vi "AppLauncher.vi"() -> ()   [LabVIEW 2016, in "Instrument.Example.lvclass"]
uses:
  Instrument.Example.lvclass
  <vilib>/JKI/JKI SMO/SMO/Typedefs/SMOState --Enum.ctl
  C:/Program Files (x86)/National Instruments/LabVIEW 2016/vi.lib/JKI/JKI SMO/SMO/SMO.lvclass
  C:/Program Files (x86)/National Instruments/LabVIEW 2016/user.lib/LevyLab/Levylab Instruments/SMOs/Instrument/Instrument.lvclass
  Instrument.Example UI/Instrument.Example UI.lvclass
  C:/Program Files (x86)/National Instruments/LabVIEW 2016/vi.lib/JKI/JKI SMO/SMO.UI/SMO.UI.lvclass
  <vilib>/JKI/JKI SMO/SMO/SMO.lvclass
  <vilib>/JKI/JKI SMO/SMO.UI/SMO.UI.lvclass
  <vilib>/Utility/sysdir.llb/System Directory Type.ctl
panel:
  out "Hardware Address":string
  out "UI SMO State":T1
  out "SMO State":T1
  out "error out":errorcluster
  in  "Stop":bool
  # "Instrument.SR7270 SMO Launcher"
  # "For instructions on how to use the JKI State Machine Objects, examples and video tutorials, visit:\nhttp://jki.net/state-machine-objects/\n\nJKI State Machine Objects™\nhttp://jki.net/state-machine-objects/\nCopyright (C) 2005-2015, JKI <info@jki.net>\nALL RIGHTS RESERVED"
  # "Starting Example Instrument..."
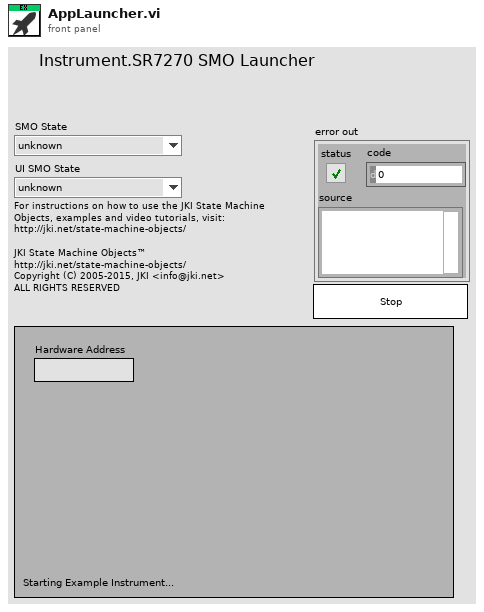
[diagram p1: front panel]
types:
  T1 = typedef "SMO.lvclass/SMOState --Enum.ctl" = enum16{"unknown", "Created", "Started", "Stopped"}
  T2 = typedef "System Directory Type.ctl" = i32
  T3 = typedef "SMO.lvclass/Public Events.ctl" = cluster{"Error":refnum<user-event>, "State":refnum<user-event>, "Reserve State":refnum<user-event>}
  T4 = cluster{"Event Registration Refnum":refnum<event-registration>, "Event Registration Refnum":refnum<event-registration>}
  T5 = enum32{"Invalid", "Standard", "Closed", "Hidden", "Minimized", "Maximized"}
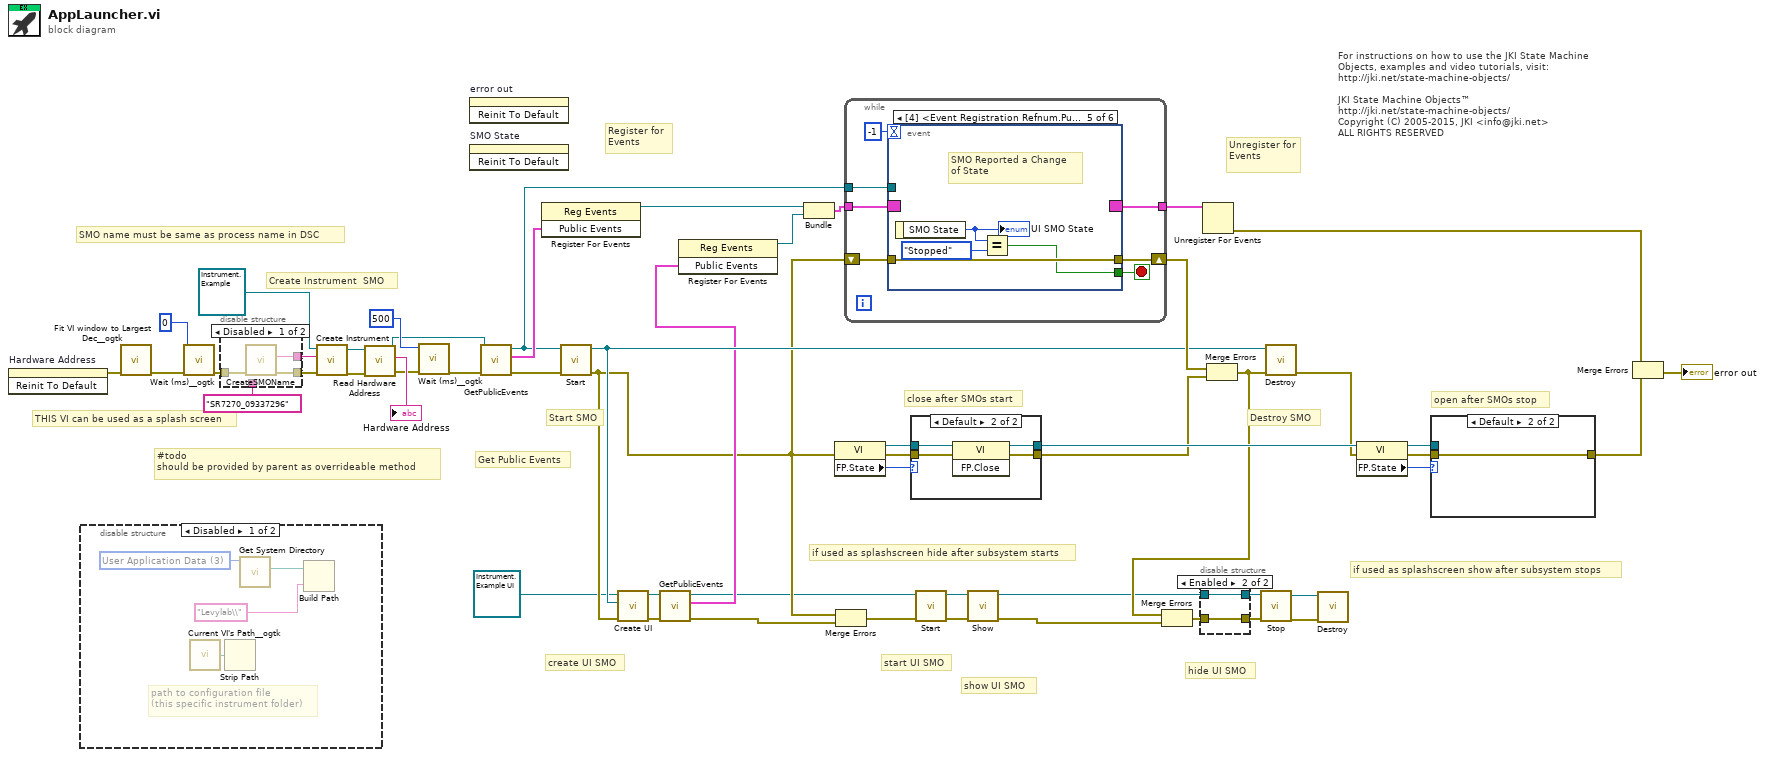
[diagram p0: block diagram]
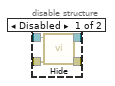
[diagram p3: hidden frame]
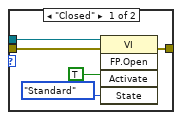
[diagram p4: hidden frame]
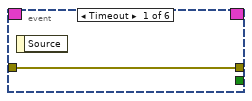
[diagram p6: hidden frame]
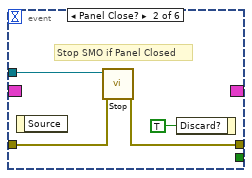
[diagram p7: hidden frame]
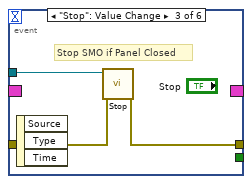
[diagram p8: hidden frame]
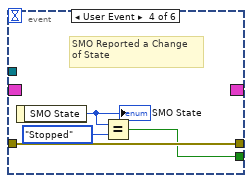
[diagram p9: hidden frame]
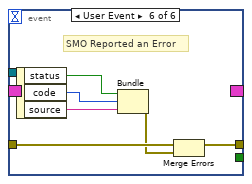
[diagram p10: hidden frame]
diagram:
  # "#todo\nshould be provided by parent as overrideable method"
  # "open after SMOs stop"
  # "close after SMOs start"
  # "hide UI SMO"
  # "show UI SMO"
  # "start UI SMO"
  # "create UI SMO"
  # "if used as splashscreen show after subsystem stops"
  # "if used as splashscreen hide after subsystem starts"
  # "THIS VI can be used as a splash screen"
  # "SMO name must be same as process name in DSC"
  # "Get Public Events"
  # "Start SMO"
  # "Destroy SMO"
  # "Create Instrument  SMO"
  # "Unregister for Events"
  # "Register for Events"
  # "For instructions on how to use the JKI State Machine Objects, examples and video tutorials, visit:\nhttp://jki.net/state-machine-objects/\n\nJKI State Machine Objects™\nhttp://jki.net/state-machine-objects/\nCopyright (C) 2005-2015, JKI <info@jki.net>\nALL RIGHTS RESERVED"
  n1 = invoke on="Hardware Address" class="Str" method="Reinit To Default"() -> (error out=w3:errorcluster)  [unwired: 3 in, 2 out]
  n2 = disable-structure shown="Disabled" {
    frame Disabled {
      w57 = T2 3 items=["User Home"=0, "User Desktop"=1, "User Documents"=2, "User Application Data"=3, "User Preferences"=4, "User Temporary"=5, "Public Documents"=6, "Public Application Data"=7, "Public Preferences"=8, "Public Cache"=13, "System Core Libraries"=9, "System Installed Libraries"=10, "Application Files"=11, "Boot Volume Root"=12] ("system directory type")
      # "path to configuration file\n(this specific instrument folder)"
      n3 = call <userlib>:"Current VI's Path__ogtk.vi"() -> ("Current VI's Path (+ Relative)"=w58:path)  [unwired: 1 in]
      n4 = Strip Path(path=w58) -> ()  [unwired: 2 out]
      n5 = call <vilib>:"Get System Directory.vi"("system directory type"=w57) -> ("system directory"=w56:path)  [unwired: 10 in]
      n6 = Build Path(base path=w56, name or relative path="Levylab\\") -> ()  [unwired: 1 out]
    }
    frame Enabled {
    }
  }
  n7 = call <userlib>:"Fit VI window to Largest Dec__ogtk.vi"("error in (no error)"=w3) -> ("error out"=w43:errorcluster)  [unwired: 5 in, 1 out]
  n8 = call <userlib>:"Wait (ms)__ogtk.vi"("error in (no error)"=w43, "milliseconds to wait"=u32 0) -> ("error out"=w13:errorcluster)  [unwired: 8 in, 1 out]
  n9 = disable-structure shown="Disabled" {
    disable-tunnel: w13 -> [w61 w62]
    disable-tunnel: [w60 w63] -> w12
    disable-tunnel: [w59 w62] -> w11
    disable-tunnel: "SR7270_09337296" ("Name") -> [_ w63]
    frame Disabled {
      n10 = call "CreateSMOName.vi"("error in (no error)"=w61) -> ("error out"=w59:errorcluster, "Name"=w60:string)  [unwired: 9 in]
    }
    frame Enabled {
    }
  }
  n11 = call-dynamic "Create Instrument.vi"("error in (no error)"=w11, "name"=w12, "Instrument in"=refnum<class "Instrument.Example.lvclass"> refnum ("Instrument.SR7270.lvclass")) -> ("error out"=w9:errorcluster, "Instrument out"=w6:refnum<class "Instrument.Example.lvclass">)  [unwired: 7 in]
  n12 = call-dynamic "Read Hardware Address.vi"("error in (no error)"=w9, "Instrument in"=w6) -> ("error out"=w8:errorcluster, "Hardware Address"=→"Hardware Address":string, "Instrument out"=w5:refnum<class "Instrument.Example.lvclass">)  [unwired: 7 in]
  n13 = call <userlib>:"Wait (ms)__ogtk.vi"("error in (no error)"=w8, "milliseconds to wait"=u32 500) -> ("error out"=w4:errorcluster)  [unwired: 8 in, 1 out]
  n14 = invoke on="error out" class="Clust (strict)" method="Reinit To Default"() -> ()  [unwired: 3 in, 3 out]
  n15 = invoke on="SMO State" class="Enum (strict)" method="Reinit To Default"() -> ()  [unwired: 3 in, 3 out]
  n16 = call <vilib>:"GetPublicEvents.vi"("error in (no error)"=w4, "SMO"=w5) -> ("error out"=w49:errorcluster, "Public Events"=w51:T3, "SMO out"=w50:refnum<class "Instrument.Example.lvclass">)  [unwired: 7 in]
  n17 = register-events(w51) -> (reference out=w42:refnum<event-registration>)  [unwired: 2 in, 1 out]
  n18 = call <vilib>:"Start.vi"("error in (no error)"=w49, "SMO"=w50) -> ("error out"=w35:errorcluster, "SMO out"=w40:refnum<class "Instrument.Example.lvclass">)  [unwired: 8 in]
  n19 = call "Create UI.vi"("error in (no error)"=w35, "Instrument.Example in"=w40, "Instrument.Example UI in"=refnum<class "Instrument.Example UI.lvclass"> refnum ("SR7220 UI.lvclass")) -> ("error out"=w38:errorcluster, "Instrument.Example UI out"=w37:refnum<class "Instrument.Example UI.lvclass">)  [unwired: 7 in]
  n20 = call <vilib>:"GetPublicEvents.vi"("error in (no error)"=w38, "SMO"=w37) -> ("error out"=w29:errorcluster, "Public Events"=w36:T3, "SMO out"=w30:refnum<class "Instrument.Example UI.lvclass">)  [unwired: 7 in]
  n21 = register-events(w36) -> (reference out=w39:refnum<event-registration>)  [unwired: 2 in, 1 out]
  n22 = Bundle("Event Registration Refnum"=w42, "Event Registration Refnum"=w39) -> (w41:T4)  [unwired: 1 in]
  n23 = property class="VI"(error in=w35) -> (reference out=w18:refnum<vi>, error out=w19:errorcluster, "FP.State"=w17:T5)  [unwired: 1 in]
  n24 = Merge Errors(w35, w29) -> (w34:errorcluster)
  n25 = while {
    shift-right: [w69] -> w48
    shift-left: w35 -> [w68]
    tunnel: w41 -> [w67]
    tunnel: [w66] -> w54
    tunnel: w50 -> [w65]
    stop <- w70 stop-if-true
    n26 = event shown="[4] <Event Registration Refnum.Public Events.State>: User Event" {
      selector: w67 -> [_ _ _ _ _ _]
      dyn-events: [_ _ _ _ _ _] -> w66
      timeout: -1 -> [_ _ _ _ _ _]
      tunnel: [_ _ _ w79 w83 _] -> w70
      tunnel: w65 -> [_ w75 w78 _ _ _]
      tunnel: [w71 w74 w77 w82 w86 w90] -> w69
      tunnel: w68 -> [w71 w73 w76 w82 w86 w88]
      event Timeout {
        n27 = event-data() -> ()  [unwired: 1 in, 1 out]
      }
      event Panel Close? {
        # "Stop SMO if Panel Closed"
        n28 = event-data() -> ()  [unwired: 1 in, 1 out]
        n29 = call <vilib>:"Stop.vi"("error in (no error)"=w73, "SMO"=w75) -> ("error out"=w74:errorcluster)  [unwired: 8 in, 1 out]
        n30 = event-data("Discard?"=TRUE ("OK")) -> ()  [unwired: 1 in, 1 out]
      }
      event "Stop": Value Change {
        # "Stop SMO if Panel Closed"
        n31 = event-data() -> ()  [unwired: 1 in, 3 out]
        n32 = call <vilib>:"Stop.vi"("error in (no error)"=w76, "SMO"=w78) -> ("error out"=w77:errorcluster)  [unwired: 8 in, 1 out]
      }
      event User Event {
        # "SMO Reported a Change\nof State"
        n33 = event-data() -> ("SMO State"=w81:T1)  [unwired: 1 in]
        "SMO State" <- w81
        n34 = Equal?(x=w81, y=SMOState_--Enum."Stopped") -> (x = y?=w79:bool)
      }
      event User Event {
        # "SMO Reported a Change\nof State"
        n35 = event-data() -> ("SMO State"=w85:T1)  [unwired: 1 in]
        "UI SMO State" <- w85
        n36 = Equal?(x=w85, y=SMOState_--Enum."Stopped") -> (x = y?=w83:bool)
      }
      event User Event {
        # "SMO Reported an Error"
        n37 = event-data() -> ("status"=w89:bool, "code"=w92:i32, "source"=w91:string)  [unwired: 1 in]
        n38 = Bundle("status"=w89, "code"=w92, "source"=w91) -> (w87:errorcluster)  [unwired: 1 in]
        n39 = Merge Errors(w88, w87) -> (w90:errorcluster)
      }
    }
  }
  n40 = case shown="Default" w17 {
    tunnel: [w94 w98] -> w44
    tunnel: w19 -> [w94 w97]
    tunnel: w18 -> [w93 w96]
    tunnel: [w93 w95] -> w47
    frame "Invalid", "Closed" {
    }
    frame Default {
      n41 = invoke class="VI" method="FP.Close"(reference=w96, error in=w97) -> (reference out=w95:refnum<vi>, error out=w98:errorcluster)  [unwired: 1 in, 1 out]
    }
  }
  n42 = call <vilib>:"Start.vi"("error in (no error)"=w34, "SMO"=w30) -> ("error out"=w28:errorcluster, "SMO out"=w27:refnum<class "Instrument.Example UI.lvclass">)  [unwired: 8 in]
  n43 = call <vilib>:"Show.vi"("error in (no error)"=w28, "SMO.UI"=w27) -> ("error out"=w26:errorcluster, "SMO.UI out"=w22:refnum<class "Instrument.Example UI.lvclass">)  [unwired: 8 in]
  n44 = Unregister For Events(event registration refnum=w54) -> (error out=w53:errorcluster)  [unwired: 1 in]
  n45 = Merge Errors(w48, w44) -> (w31:errorcluster)
  n46 = Merge Errors(w31, w26) -> (w23:errorcluster)
  n47 = disable-structure shown="Enabled" {
    disable-tunnel: [w102 w103] -> w25
    disable-tunnel: [w101 w104] -> w24
    disable-tunnel: w23 -> [w100 w103]
    disable-tunnel: w22 -> [w99 w104]
    frame Disabled {
      n48 = call <vilib>:"Hide.vi"("error in (no error)"=w100, "SMO.UI"=w99) -> ("error out"=w102:errorcluster, "SMO.UI out"=w101:refnum<class "Instrument.Example UI.lvclass">)  [unwired: 8 in]
    }
    frame Enabled {
    }
  }
  n49 = call <vilib>:"Stop.vi"("error in (no error)"=w25, "SMO"=w24) -> ("error out"=w33:errorcluster, "SMO out"=w32:refnum<class "Instrument.Example UI.lvclass">)  [unwired: 8 in]
  n50 = call <vilib>:"Destroy.vi"("error in (no error)"=w31, "SMO"=w40) -> ("error out"=w46:errorcluster)  [unwired: 9 in]
  n51 = call <vilib>:"Destroy.vi"("error in (no error)"=w33, "SMO"=w32) -> ()  [unwired: 9 in, 1 out]
  n52 = property class="VI"(reference=w47, error in=w46) -> (reference out=w15:refnum<vi>, error out=w16:errorcluster, "FP.State"=w14:T5)
  n53 = case shown="Default" w14 {
    tunnel: [w107 w110] -> w45
    tunnel: w16 -> [w106 w110]
    tunnel: w15 -> [w105 _]
    frame "Closed" {
      n54 = invoke class="VI" method="FP.Open"(reference=w105, error in=w106, "Activate"=TRUE, "State"=T5."Standard") -> (error out=w107:errorcluster)  [unwired: 1 in, 4 out]
    }
    frame Default {
    }
  }
  n55 = Merge Errors(w53, w45) -> (→"error out":errorcluster)
